vi "MAIN FPGA V2.vi"() -> ()   [LabVIEW 2019]
uses:
  TypeDef/FPGA AIs.ctl
  TypeDef/FPGA AI Loop Data.ctl
  TypeDef/FPGA DO Loop Data.ctl
  TypeDef/FPGA DI Loop Data.ctl
  TypeDef/DO index.ctl
  <vilib>/rvi/Emulation/niFpgaGetClockAttributes.vi
  <vilib>/rvi/Emulation/niFpgaSctlEmulationGetInTimedLoop.vi
  <vilib>/rvi/Emulation/niFpgaEmulationReportErrorSimple.vi
  <vilib>/rvi/interface/RandomDataEmulation/niFpgaRandomDataHandleErrors.vi
  <vilib>/rvi/Emulation/niFpgaEmulationIsFPGAContextNoSignature.vi
  <vilib>/rvi/errors/niFpgaSetErrorForExecOnDevCompSimple.vi
  <vilib>/rvi/eio/common/nirviEmuReportErrorAndStop.vi
  <vilib>/rvi/DataTransferAndStorage/Container/Common/niFpgaContainerGetUniqueNameForEmu.vi
  <vilib>/rvi/FIFO/Fifo_Resource/nirvififoEmulationSetSize.vi
  <vilib>/rvi/FIFO/Fifo_Resource/nirviFifoEmulationQueueMgr.vi
  <instcachedir>/0/nirviFifoEmulationQueueMgr_E5CAEC123FF24DC58D834DCA3CDAA9B5.lvgen/nirviFifoEmulationQueueMgr_E5CAEC123FF24DC58D834DCA3CDAA9B5_002.vi
  <vilib>/rvi/FIFO/Fifo_Resource/nirvififoEmulationDetermineInputValidOut.vi
  <vilib>/rvi/FIFO/Fifo_Resource/nirvififoEmulationCreateLock.vi
  <vilib>/rvi/Emulation/niFpgaProcessEmulError.vi
  <vilib>/rvi/FIFO/Fifo_Resource/nirvififoEmulationObtainLock.vi
  <vilib>/rvi/FIFO/Fifo_Resource/nirvififoEmulationReleaseLock.vi
  <vilib>/rvi/occurrence/nirviWaitOnOccurrenceBase.vi
  <vilib>/rvi/errors/nirviReportUnexpectedCaseInternalError.vi
  <vilib>/rvi/errors/nirviReportUnexpectedCaseInternalError (U32).vi
  <vilib>/rvi/Emulation/niFpgaCriticalErrorInLSC.vi
  <vilib>/rvi/eio/common/nirviEmuTemplateMethod_errors.vi
  <vilib>/rvi/DataTransferAndStorage/Container/XNode/niFpgaContainer.xnode
  <vilib>/rvi/interface/RandomDataEmulation/nirviRandomDataFpgaReadWriteTemplate.vi
  <vilib>/rvi/FIFO/Fifo_Resource/nirvififoEmulationWrite.vi
  <vilib>/eio/EIONode/EIONode.xnode
panel:
  out "DO":u32
  out "Discrete Control Filter":T1
  out "Average 1ms":T1
  out "Raw":T1
  in  "Cycles to Filter AI":u16=2
  in  "Enable Close Inlet":bool
  in  "SP Close Inlet":fxp<+/-,21,-4>
  in  "Enable Close Outlet":bool
  in  "SP Close Outlet":fxp<+/-,21,-4>
  in  "Enable Stop Drive":bool
  in  "SP Stop Drive":fxp<+/-,21,-4>
  out "Error AO":errorcluster
  in  "Mod5/AO0":fxp<+/-,20,5>
  in  "Mod5/AO1":fxp<+/-,20,5>
  in  "Mod5/AO2":fxp<+/-,20,5>
  in  "Mod5/AO3":fxp<+/-,20,5>
  out "dt (ticks) AO Loop":u32
  out "DI":u32
  out "Error DI":errorcluster
  in  "Cycles to Filter":u16=100
  out "dt(tiks) DI loop":u32
  out "Error DO":errorcluster
  out "FIFO AI Timed Out?":bool
  out "Error AI mod 2":errorcluster
  out "Error AI mod 1":errorcluster
  out "dt(tiks) DO loop":u32
  out "dt(tiks) AI loop":u32
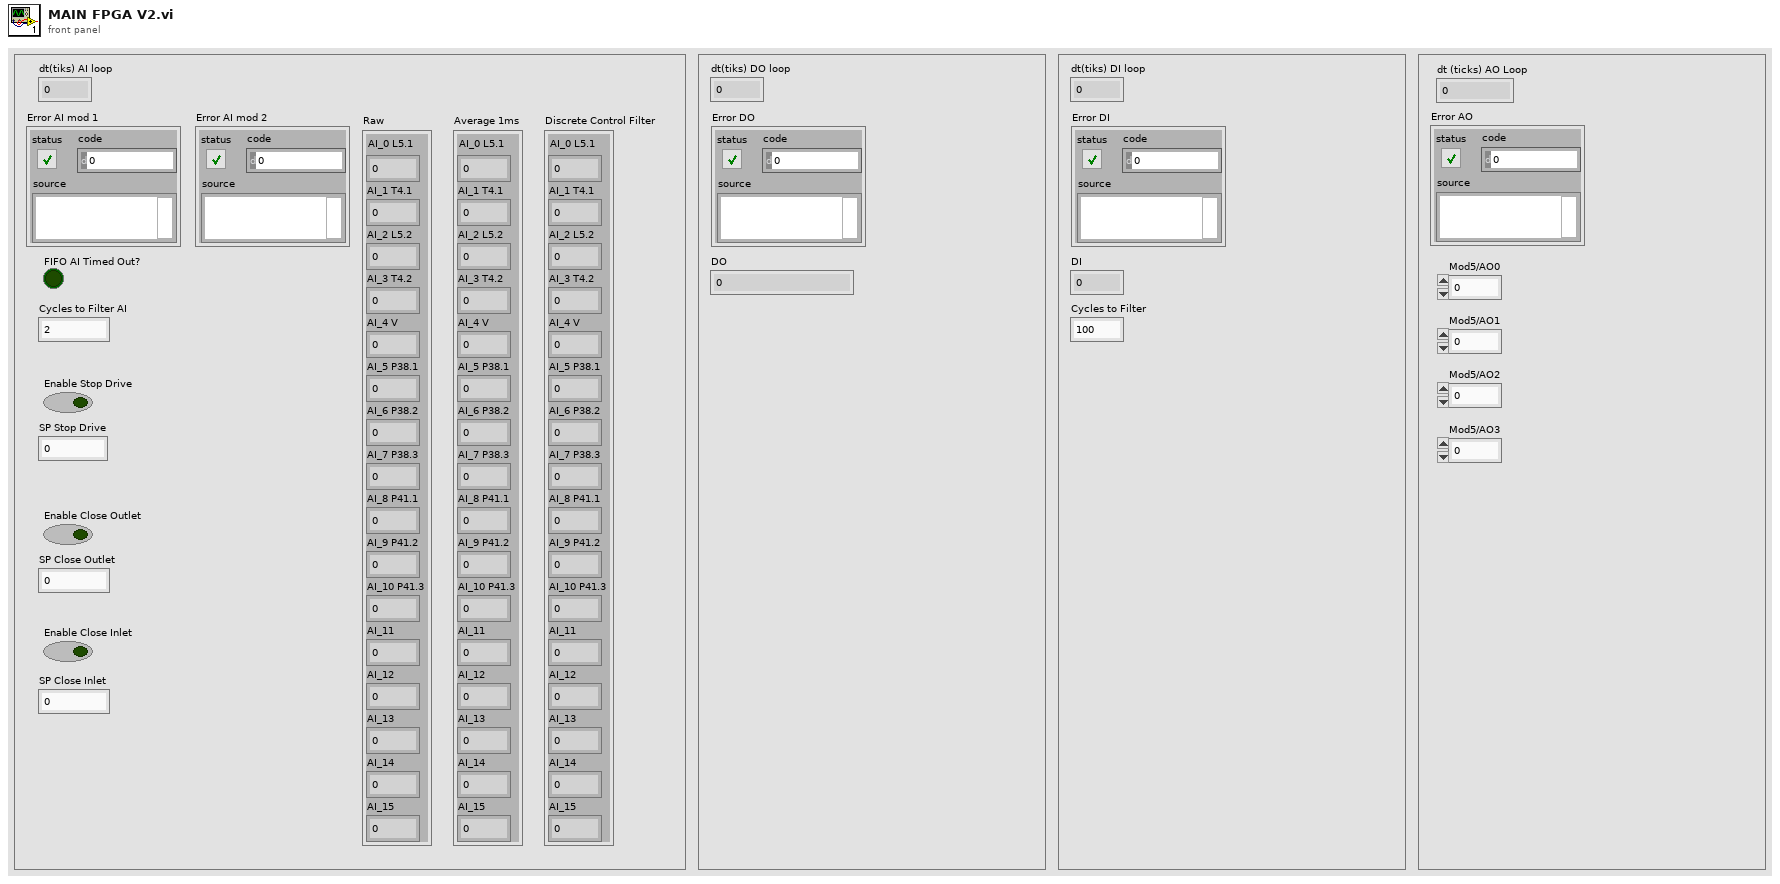
[diagram p1: front panel]
types:
  T1 = typedef "FPGA AIs.ctl" = cluster{"AI_0 L5.1":fxp<+/-,21,-4>, "AI_1 T4.1":fxp<+/-,21,-4>, "AI_2 L5.2":fxp<+/-,21,-4>, "AI_3 T4.2":fxp<+/-,21,-4>, "AI_4 V":fxp<+/-,21,-4>, "AI_5 P38.1":fxp<+/-,21,-4>, "AI_6 P38.2":fxp<+/-,21,-4>, "AI_7 P38.3":fxp<+/-,21,-4>, "AI_8 P41.1":fxp<+/-,21,-4>, "AI_9 P41.2":fxp<+/-,21,-4>, "AI_10 P41.3":fxp<+/-,21,-4>, "AI_11":fxp<+/-,21,-4>, "AI_12":fxp<+/-,21,-4>, "AI_13":fxp<+/-,21,-4>, "AI_14":fxp<+/-,21,-4>, "AI_15":fxp<+/-,21,-4>}
  T2 = typedef "FPGA DI Loop Data.ctl" = cluster{"DI":bool[], "Set Time uSec":u16[]}
  T3 = typedef "FPGA DO Loop Data.ctl" = cluster{"DO":bool[], "Is Pulse":bool[], "Set Time uSec":u32[], "Wait Time uSec":u32[]}
  T4 = typedef "FPGA AI Loop Data.ctl" = cluster{"Raw":T1, "Average 1ms":T1, "Discrete Control Filter":T1, "mean valid":bool}
  T5 = typedef "DO index.ctl" = u8
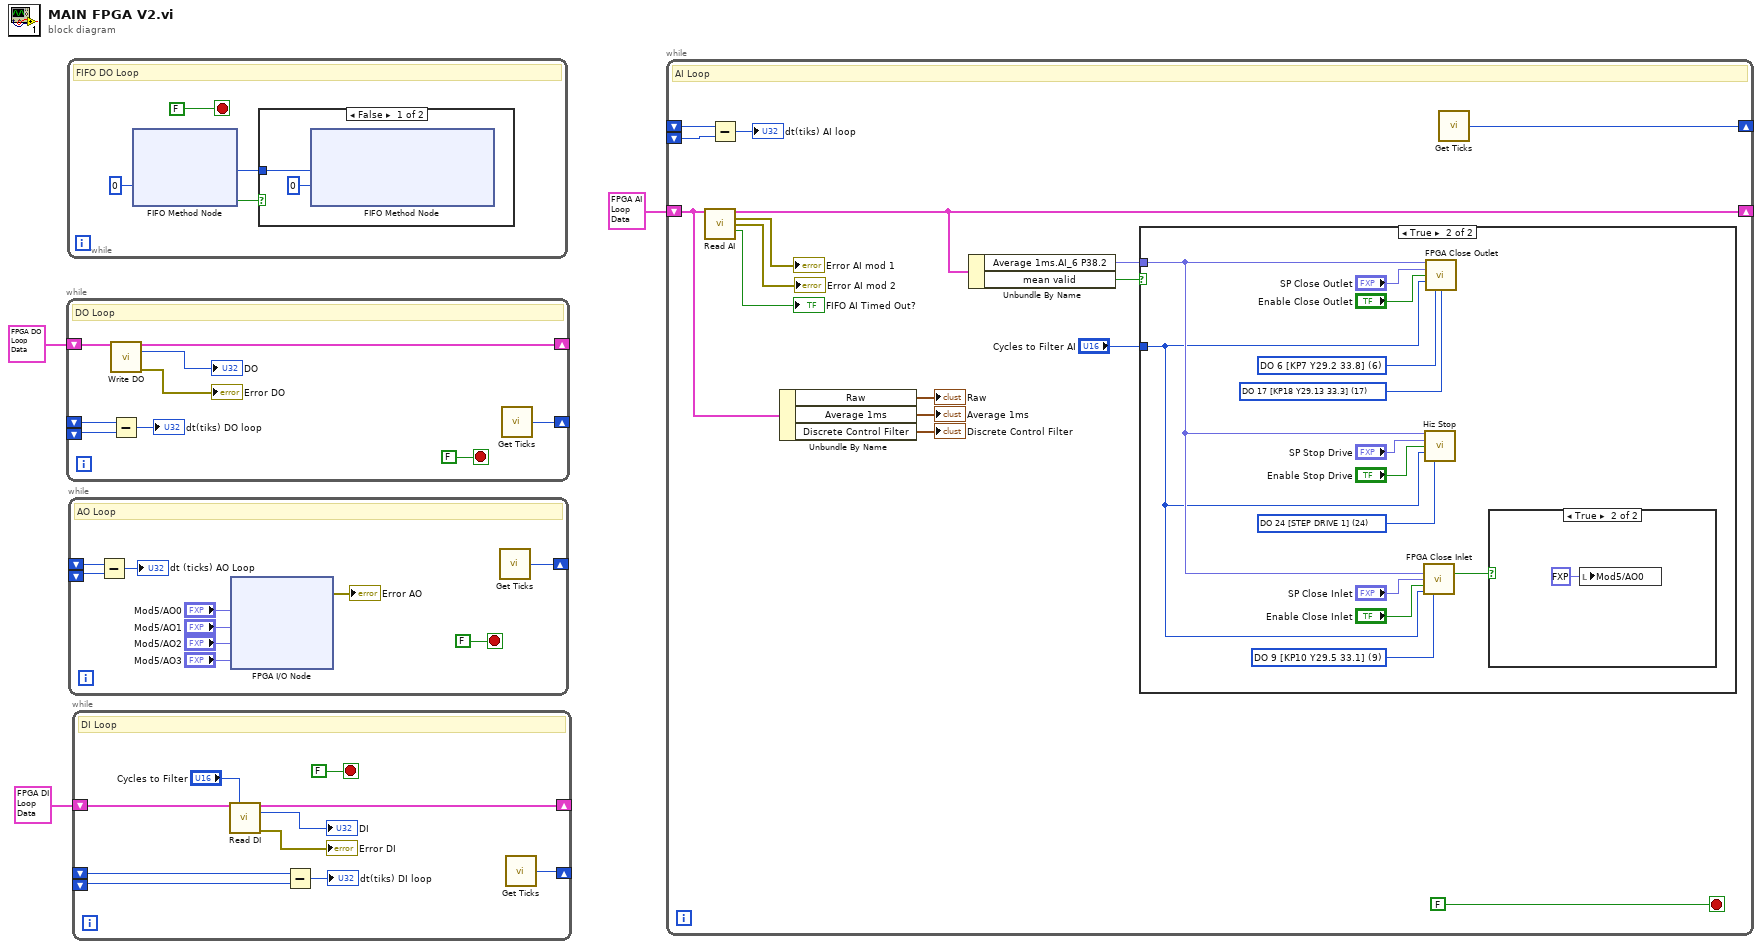
[diagram p0: block diagram]
diagram:
  n1 = while {
    shift-right: [w7] -> _
    shift-left: T3 {"DO"=[FALSE, FALSE, FALSE, FALSE, FALSE, FALSE, FALSE, FALSE, FALSE, FALSE, FALSE, FALSE, FALSE, FALSE, FALSE, FALSE, FALSE, FALSE, FALSE, FALSE, FALSE, FALSE, FALSE, FALSE, FALSE, FALSE, FALSE, FALSE, FALSE, FALSE, FALSE, FALSE], "Is Pulse"=[FALSE, FALSE, FALSE, FALSE, FALSE, FALSE, FALSE, FALSE, FALSE, FALSE, FALSE, FALSE, FALSE, FALSE, FALSE, FALSE, FALSE, FALSE, FALSE, FALSE, FALSE, FALSE, FALSE, FALSE, FALSE, FALSE, FALSE, FALSE, FALSE, FALSE, FALSE, FALSE], "Set Time uSec"=[0, 0, 0, 0, 0, 0, 0, 0, 0, 0, 0, 0, 0, 0, 0, 0, 0, 0, 0, 0, 0, 0, 0, 0, 0, 0, 0, 0, 0, 0, 0, 0], "Wait Time uSec"=[0, 0, 0, 0, 0, 0, 0, 0, 0, 0, 0, 0, 0, 0, 0, 0, 0, 0, 0, 0, 0, 0, 0, 0, 0, 0, 0, 0, 0, 0, 0, 0]} ("FPGA DO Loop Data") -> [w8]
    shift-right: [w5] -> _
    shift-left: _ -> [w10]
    shift-left: _ -> [w9]
    stop <- FALSE stop-if-true
    # "DO Loop"
    n2 = call "Write DO.vi"("FPGA DO Loop Data in"=w8) -> ("FPGA DO Loop Data out"=w7:T3, "DO"=→"DO":u32, "error out"=→"Error DO":errorcluster)  [unwired: 12 in]
    n3 = Subtract(x=w10, y=w9) -> (x-y=→"dt(tiks) DO loop":u32)
    n4 = call "Get Ticks.vi"() -> ("Tick Count(Ticks)"=w5:u32)
  }
  n5 = while {
    stop <- FALSE stop-if-true
    # "FIFO DO Loop"
    n6 = xnode ("FIFO Method Node")("Timeout"=0) -> ("Element"=w13:u64, "Timed Out?"=w14:bool)  [unwired: 1 in, 1 out]
    n7 = case shown="False" w14 {
      tunnel: w13 -> [w18 _]
      frame False {
        n8 = xnode ("FIFO Method Node")("Element"=w18, "Timeout"=0) -> ()  [unwired: 1 in, 2 out]
      }
      frame True {
      }
    }
  }
  n9 = while {
    shift-right: [w19] -> _
    shift-left: _ -> [w21]
    shift-left: _ -> [w20]
    stop <- FALSE stop-if-true
    # "AO Loop"
    n10 = Subtract(x=w21, y=w20) -> (x-y=→"dt (ticks) AO Loop":u32)
    n11 = xnode "FPGA I/O Node"("Mod5/AO0"="Mod5/AO0", "Mod5/AO1"="Mod5/AO1", "Mod5/AO2"="Mod5/AO2", "Mod5/AO3"="Mod5/AO3") -> ("error out"=→"Error AO":errorcluster)  [unwired: 5 in, 4 out]
    n12 = call "Get Ticks.vi"() -> ("Tick Count(Ticks)"=w19:u32)
  }
  n13 = while {
    shift-right: [w33] -> _
    shift-left: T2 {"DI"=[FALSE, FALSE, FALSE, FALSE, FALSE, FALSE, FALSE, FALSE, FALSE, FALSE, FALSE, FALSE, FALSE, FALSE, FALSE, FALSE, FALSE, FALSE, FALSE, FALSE, FALSE, FALSE, FALSE, FALSE, FALSE, FALSE, FALSE, FALSE, FALSE, FALSE, FALSE, FALSE], "Set Time uSec"=[0, 0, 0, 0, 0, 0, 0, 0, 0, 0, 0, 0, 0, 0, 0, 0, 0, 0, 0, 0, 0, 0, 0, 0, 0, 0, 0, 0, 0, 0, 0, 0]} ("FPGA DI Loop Data") -> [w37]
    shift-right: [w29] -> _
    shift-left: _ -> [w35]
    shift-left: _ -> [w34]
    stop <- FALSE stop-if-true
    # "DI Loop"
    n14 = call "Read DI.vi"("FPGA DI Loop Data in"=w37, "Cycles to Filter"="Cycles to Filter") -> ("FPGA DI Loop Data out"=w33:T2, "DI"=→"DI":u32, "error out"=→"Error DI":errorcluster)  [unwired: 11 in]
    n15 = Subtract(x=w35, y=w34) -> (x-y=→"dt(tiks) DI loop":u32)
    n16 = call "Get Ticks.vi"() -> ("Tick Count(Ticks)"=w29:u32)
  }
  n17 = while {
    shift-right: [w47] -> _
    shift-left: T4 {"Raw"={"AI_0 L5.1"=0.0, "AI_1 T4.1"=0.0, "AI_2 L5.2"=0.0, "AI_3 T4.2"=0.0, "AI_4 V"=0.0, "AI_5 P38.1"=0.0, "AI_6 P38.2"=0.0, "AI_7 P38.3"=0.0, "AI_8 P41.1"=0.0, "AI_9 P41.2"=0.0, "AI_10 P41.3"=0.0, "AI_11"=0.0, "AI_12"=0.0, "AI_13"=0.0, "AI_14"=0.0, "AI_15"=0.0}, "Average 1ms"={"AI_0 L5.1"=0.0, "AI_1 T4.1"=0.0, "AI_2 L5.2"=0.0, "AI_3 T4.2"=0.0, "AI_4 V"=0.0, "AI_5 P38.1"=0.0, "AI_6 P38.2"=0.0, "AI_7 P38.3"=0.0, "AI_8 P41.1"=0.0, "AI_9 P41.2"=0.0, "AI_10 P41.3"=0.0, "AI_11"=0.0, "AI_12"=0.0, "AI_13"=0.0, "AI_14"=0.0, "AI_15"=0.0}, "Discrete Control Filter"={"AI_0 L5.1"=0.0, "AI_1 T4.1"=0.0, "AI_2 L5.2"=0.0, "AI_3 T4.2"=0.0, "AI_4 V"=0.0, "AI_5 P38.1"=0.0, "AI_6 P38.2"=0.0, "AI_7 P38.3"=0.0, "AI_8 P41.1"=0.0, "AI_9 P41.2"=0.0, "AI_10 P41.3"=0.0, "AI_11"=0.0, "AI_12"=0.0, "AI_13"=0.0, "AI_14"=0.0, "AI_15"=0.0}, "mean valid"=FALSE} ("FPGA AI Loop Data in") -> [w44]
    shift-right: [w40] -> _
    shift-left: _ -> [w53]
    shift-left: _ -> [w52]
    stop <- FALSE stop-if-true
    # "AI Loop"
    n18 = call "Read AI.vi"("FPGA AI Loop Data in"=w44) -> ("FPGA AI Loop Data out"=w47:T4, "Error AI mod 1"=→"Error AI mod 1":errorcluster, "Error AI mod 2"=→"Error AI mod 2":errorcluster, "FIFO AI Timed Out?"=→"FIFO AI Timed Out?":bool)  [unwired: 11 in]
    n19 = Subtract(x=w53, y=w52) -> (x-y=→"dt(tiks) AI loop":u32)
    n20 = Unbundle By Name(w44) -> ("Raw"=→"Raw":T1, "Average 1ms"=→"Average 1ms":T1, "Discrete Control Filter"=→"Discrete Control Filter":T1)
    n21 = Unbundle By Name(w47) -> ("Average 1ms.AI_6 P38.2"=w46:fxp<+/-,21,-4>, "mean valid"=w39:bool)
    n22 = case shown="True" w39 {
      tunnel: w46 -> [_ w60]
      tunnel: "Cycles to Filter AI" -> [_ w56]
      frame False {
      }
      frame True {
        w57 = T5 9 items=["DO 0 [KP1 [DO 0]]", "DO 1 [ON KP2 [DO 1]]", "DO 2 [ON KP3 [DO 2]]", "DO 3 [WATER Y18.1 [DO3]]", "DO 4 [WATER Y18.2 [DO4]]", "DO 5 [KP6 Y29.1 33.7]", "DO 6 [KP7 Y29.2 33.8]", "DO 7 [KP8 Y29.3 33.9]", "DO 8 [KP9 Y29.4  33.12]", "DO 9 [KP10 Y29.5 33.1]", "DO 10 [KP11 Y29.6 33.2]", "DO 11 [KP12 Y29.7  33.13]", "DO 12 [KP13 Y29.8  33.11]", "DO 13 [KP14 Y29.9 33.10]", "DO 14 [KP15 Y29.10  33.6]", "DO 15 [KP16 Y29.11  33.5]", "DO 16 [KP17 Y29.12  33.4]", "DO 17 [KP18 Y29.13 33.3]", "DO 18 [AIR KP19]", "DO 19 [STEP DRIVE EN KP20]", "DO 20 [KP21 Y44.1 OPEN]", "DO 21 [ KP22 Y44.1 CLOSE]", "DO 22 [ KP23 Y44.2 OPEN]", "DO 23", "DO 24 [STEP DRIVE 1]", "DO 25 [STEP DRIVE 2]"] ("#DO")
        w64 = T5 24 items=["DO 0 [KP1 [DO 0]]", "DO 1 [ON KP2 [DO 1]]", "DO 2 [ON KP3 [DO 2]]", "DO 3 [WATER Y18.1 [DO3]]", "DO 4 [WATER Y18.2 [DO4]]", "DO 5 [KP6 Y29.1 33.7]", "DO 6 [KP7 Y29.2 33.8]", "DO 7 [KP8 Y29.3 33.9]", "DO 8 [KP9 Y29.4  33.12]", "DO 9 [KP10 Y29.5 33.1]", "DO 10 [KP11 Y29.6 33.2]", "DO 11 [KP12 Y29.7  33.13]", "DO 12 [KP13 Y29.8  33.11]", "DO 13 [KP14 Y29.9 33.10]", "DO 14 [KP15 Y29.10  33.6]", "DO 15 [KP16 Y29.11  33.5]", "DO 16 [KP17 Y29.12  33.4]", "DO 17 [KP18 Y29.13 33.3]", "DO 18 [AIR KP19]", "DO 19 [STEP DRIVE EN KP20]", "DO 20 [KP21 Y44.1 OPEN]", "DO 21 [ KP22 Y44.1 CLOSE]", "DO 22 [ KP23 Y44.2 OPEN]", "DO 23", "DO 24 [STEP DRIVE 1]", "DO 25 [STEP DRIVE 2]"] ("DO STEP DRIVE STOP 1")
        w62 = T5 17 items=["DO 0 [KP1 [DO 0]]", "DO 1 [ON KP2 [DO 1]]", "DO 2 [ON KP3 [DO 2]]", "DO 3 [WATER Y18.1 [DO3]]", "DO 4 [WATER Y18.2 [DO4]]", "DO 5 [KP6 Y29.1 33.7]", "DO 6 [KP7 Y29.2 33.8]", "DO 7 [KP8 Y29.3 33.9]", "DO 8 [KP9 Y29.4  33.12]", "DO 9 [KP10 Y29.5 33.1]", "DO 10 [KP11 Y29.6 33.2]", "DO 11 [KP12 Y29.7  33.13]", "DO 12 [KP13 Y29.8  33.11]", "DO 13 [KP14 Y29.9 33.10]", "DO 14 [KP15 Y29.10  33.6]", "DO 15 [KP16 Y29.11  33.5]", "DO 16 [KP17 Y29.12  33.4]", "DO 17 [KP18 Y29.13 33.3]", "DO 18 [AIR KP19]", "DO 19 [STEP DRIVE EN KP20]", "DO 20 [KP21 Y44.1 OPEN]", "DO 21 [ KP22 Y44.1 CLOSE]", "DO 22 [ KP23 Y44.2 OPEN]", "DO 23", "DO 24 [STEP DRIVE 1]", "DO 25 [STEP DRIVE 2]"] ("#DO 2")
        w63 = T5 6 items=["DO 0 [KP1 [DO 0]]", "DO 1 [ON KP2 [DO 1]]", "DO 2 [ON KP3 [DO 2]]", "DO 3 [WATER Y18.1 [DO3]]", "DO 4 [WATER Y18.2 [DO4]]", "DO 5 [KP6 Y29.1 33.7]", "DO 6 [KP7 Y29.2 33.8]", "DO 7 [KP8 Y29.3 33.9]", "DO 8 [KP9 Y29.4  33.12]", "DO 9 [KP10 Y29.5 33.1]", "DO 10 [KP11 Y29.6 33.2]", "DO 11 [KP12 Y29.7  33.13]", "DO 12 [KP13 Y29.8  33.11]", "DO 13 [KP14 Y29.9 33.10]", "DO 14 [KP15 Y29.10  33.6]", "DO 15 [KP16 Y29.11  33.5]", "DO 16 [KP17 Y29.12  33.4]", "DO 17 [KP18 Y29.13 33.3]", "DO 18 [AIR KP19]", "DO 19 [STEP DRIVE EN KP20]", "DO 20 [KP21 Y44.1 OPEN]", "DO 21 [ KP22 Y44.1 CLOSE]", "DO 22 [ KP23 Y44.2 OPEN]", "DO 23", "DO 24 [STEP DRIVE 1]", "DO 25 [STEP DRIVE 2]"] ("#DO 1")
        n23 = call "FPGA Close Inlet.vi"("PV"=w60, "SP Close Inlet"="SP Close Inlet", "Enable Close Inlet"="Enable Close Inlet", "Cycles to Filter"=w56, "#DO"=w57) -> ("Close cmd"=w55:bool)  [unwired: 10 in]
        n24 = call "Hiz Stop.vi"("PV"=w60, "SP"="SP Stop Drive", "Enable Stop Drive"="Enable Stop Drive", "Cycles to Filter"=w56, "DO STEP DRIVE STOP"=w64) -> ()  [unwired: 11 in]
        n25 = call "FPGA Close Outlet.vi"("PV"=w60, "SP Close Outlet"="SP Close Outlet", "Enable Close Outlet"="Enable Close Outlet", "Cycles to Filter"=w56, "#DO 1"=w63, "#DO 2"=w62) -> ()  [unwired: 10 in]
        n26 = case shown="True" w55 {
          frame False {
          }
          frame True {
            n27 = local write "Mod5/AO0"(fxp<+/-,20,5> 0.0 ("Mod5/AO0")) -> ()
          }
        }
      }
    }
    n28 = call "Get Ticks.vi"() -> ("Tick Count(Ticks)"=w40:u32)
  }
